vi "Debouncer_Execute.vi"(5 "DebounceType":T1, 7 "DebounceTime":dbl, 8 "CurrentTIme":dbl=-1.0, 11 "Input":bool) -> (3 "Output":bool, 4 "Debouncer":T2 {"PrevTimeSeconds" format="%13.6p"; "DebounceTimeSeconds" format="%13.6p"})   [LabVIEW 2019, in "Trajectory_Library.lvlib"]
doc: "A simple debounce filter for boolean streams. Requires that the boolean change value from baseline for a specified period of time before the filtered value changes.\n\nThis is a LabVIEW style single function call.\n\nInputs:\n - DebounceType -- Which type of state change the debouncing will be performed on. (Optional: Default: Rising)\n - DebounceTime -- The number of seconds the value must change from baseline for the filtered value to change.\n - Input -- Boolean input value.\n - CurrentTime -- Current system running time. (Optional - Default: Read system time.)\n\nOutput:\n - Output -- Value of debounced input.\n - Debouncer -- Initialized data cluster for debouncer."
uses:
  Trajectory_Library.lvlib
  Enum/DEBOUNCER_TYPE_ENUM.ctl
  TypeDef/DEBOUNCER.ctl
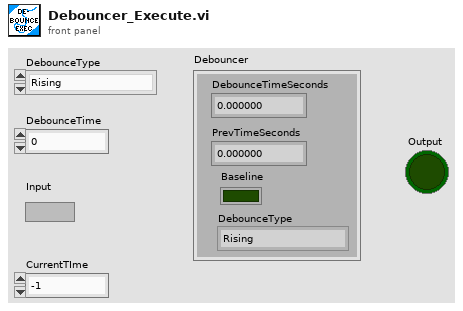
[diagram p1: front panel]
types:
  T1 = typedef "Trajectory_Library.lvlib/DEBOUNCER_TYPE_ENUM.ctl" = enum16{"Rising", "Falling", "Both"}
  T2 = typedef "Trajectory_Library.lvlib/DEBOUNCER.ctl" = cluster{"DebounceTimeSeconds":dbl, "PrevTimeSeconds":dbl, "Baseline":bool, "DebounceType":T1}
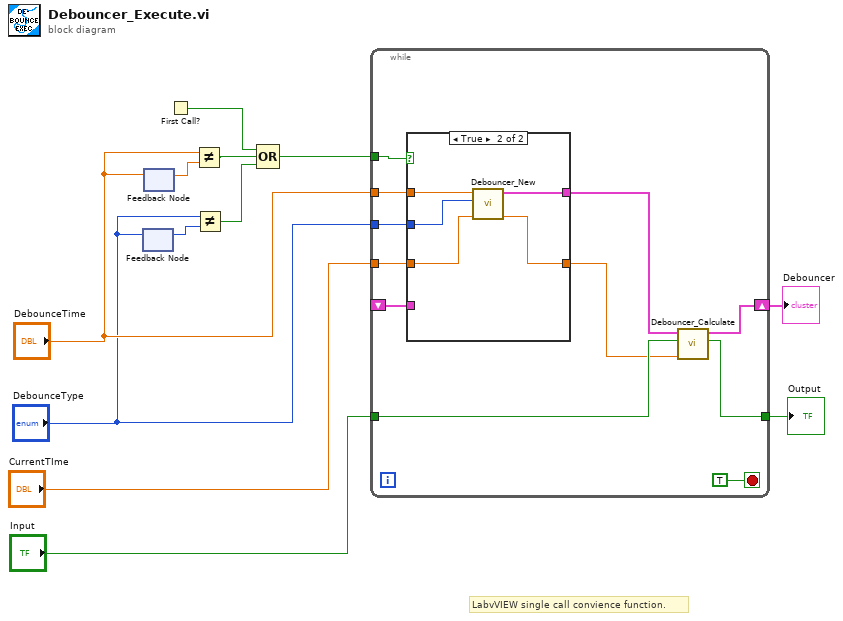
[diagram p0: block diagram]
diagram:
  # "LabvVIEW single call convience function."
  n1 = feedback-in #1("DebounceType") -> ()
  n2 = feedback #1() -> (w9:T1)  [unwired: 1 in]
  n3 = feedback #2() -> (w11:dbl)  [unwired: 1 in]
  n4 = feedback-in #2("DebounceTime") -> ()
  n5 = First Call?() -> (First Call?: T/F=w12:bool)
  n6 = Not Equal?(x="DebounceTime", y=w11) -> (x != y?=w10:bool)
  n7 = Not Equal?(x="DebounceType", y=w9) -> (x != y?=w8:bool)
  n8 = Compound Arithmetic op=OR(w12, w10, w8) -> (w7:bool)
  n9 = while {
    tunnel: w7 -> [w23]
    tunnel: "DebounceTime" -> [w22]
    tunnel: "DebounceType" -> [w21]
    tunnel: "CurrentTIme" -> [w20]
    tunnel: "Input" -> [w18]
    tunnel: [w16] -> w2
    shift-right: [w15] -> w1
    shift-left: _ -> [w14]
    stop <- TRUE stop-if-true
    n10 = case shown="True" w23 {
      tunnel: w22 -> [_ w30]
      tunnel: w21 -> [_ w29]
      tunnel: w20 -> [w25 w28]
      tunnel: [w24 w27] -> w19
      tunnel: [w25 w26] -> w17
      tunnel: w14 -> [w24 _]
      frame False {
      }
      frame True {
        n11 = call "Debouncer_New.vi"("CurrentTIme"=w28, "DebounceType"=w29, "DebounceTime"=w30) -> ("CurrentTIme Out"=w26:dbl, "Debouncer"=w27:T2)  [unwired: 7 in]
      }
    }
    n12 = call "Debouncer_Calculate.vi"("CurrentTIme"=w17, "Input"=w18, "Debouncer In"=w19) -> ("Output"=w16:bool, "Debouncer Out"=w15:T2)  [unwired: 6 in, 1 out]
  }
  "Debouncer" <- w1
  "Output" <- w2
